vi "paths.vi"() -> ()   [LabVIEW 2022 SP3]
uses:
  <vilib>/Utility/file.llb/Write Delimited Spreadsheet (string).vi
panel:
  out "Array 2":path[](array[path])
  out "filenames":string[][](array[string])
  in  "path":path=path "D:/Doppler Retro/2009"
  in  "folder names 2":string[](array[string])
  out "Array":path[](array[path])
  out "folder names":string[](array[string])
  out "All Files in Dir":path[](array[path])
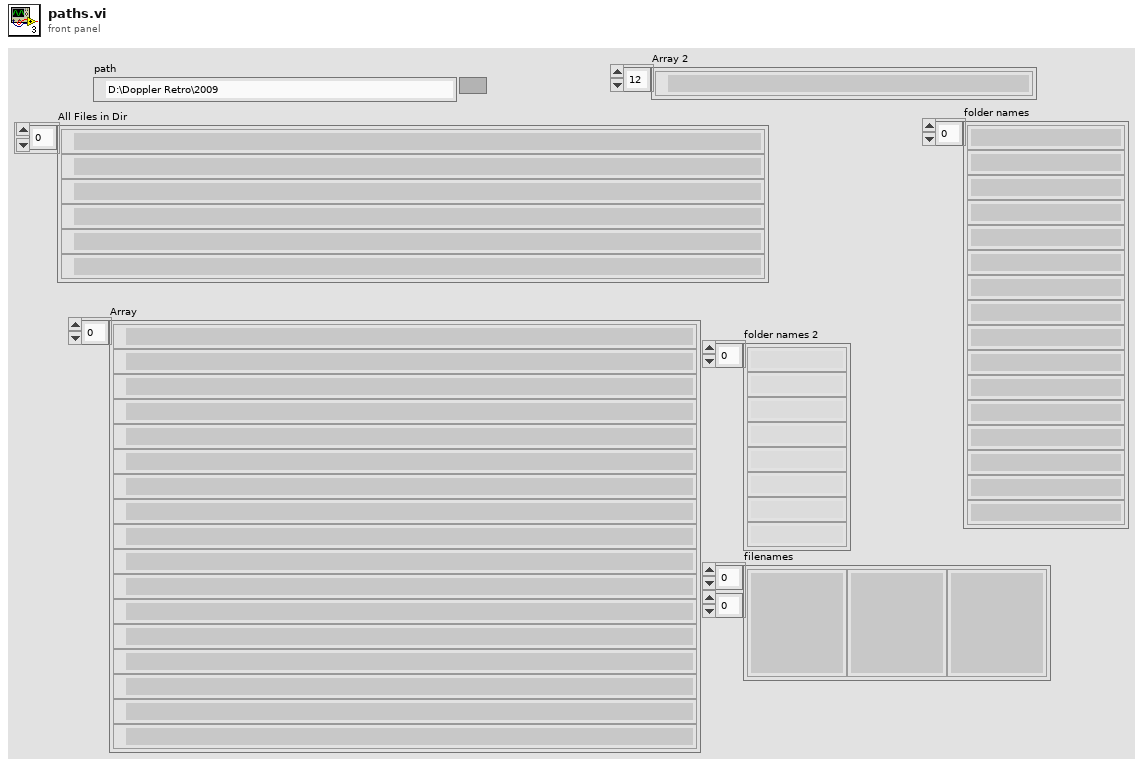
[diagram p1: front panel]
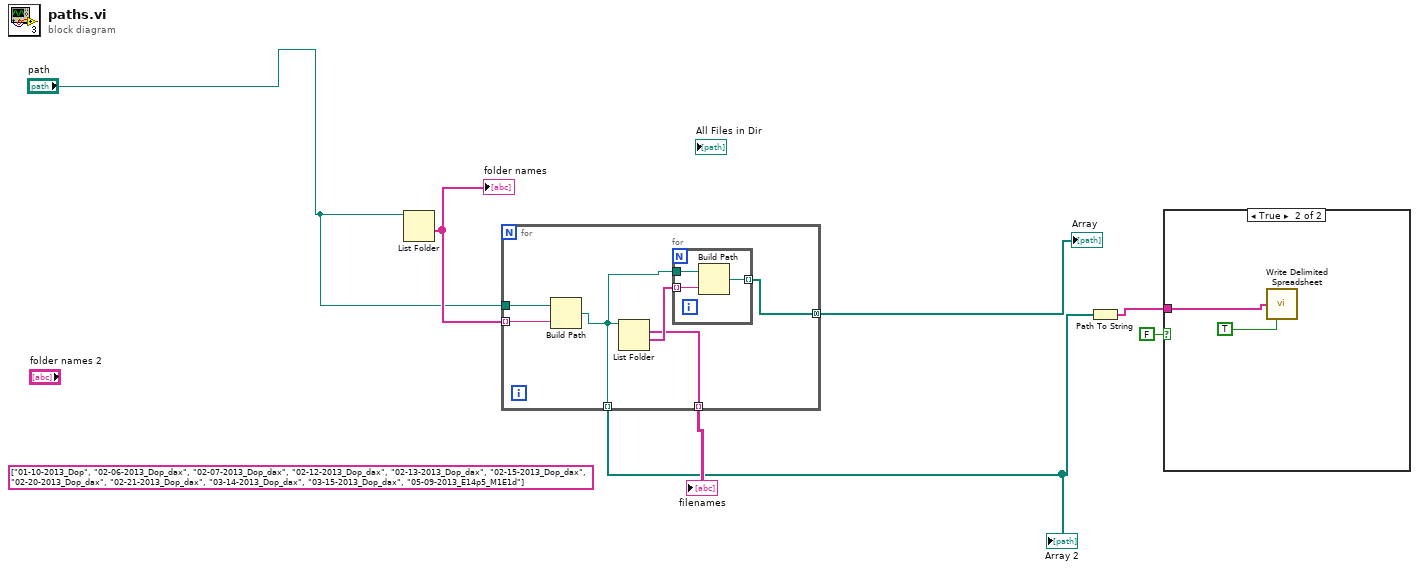
[diagram p0: block diagram]
diagram:
  (unwired) string[] ["01-10-2013_Dop", "02-06-2013_Dop_dax", "02-07-2013_Dop_dax", "02-12-2013_Dop_dax", "02-13-2013_Dop_dax", "02-15-2013_Dop_dax", "02-20-2013_Dop_dax", "02-21-2013_Dop_dax", "03-14-2013_Dop_dax", "03-15-2013_Dop_dax", "05-09-2013_E14p5_M1E1d"] ("folder names")
  n1 = List Folder(path="path") -> (folder names=w4:string[])  [unwired: 3 in, 3 out]
  "folder names" <- w4
  n2 = for {
    tunnel: "path" -> [w13]
    tunnel: w4 -> [w12] mode=indexing
    tunnel: [w10] -> w7 mode=concatenating
    tunnel: [w9] -> w2 mode=indexing
    tunnel: [w8] -> w1 mode=indexing
    n3 = Build Path(base path=w13, name or relative path=w12) -> (appended path=w8:path)
    n4 = List Folder(path=w8) -> (filenames=w9:string[], folder names=w11:string[])  [unwired: 3 in, 2 out]
    n5 = for {
      tunnel: w8 -> [w16]
      tunnel: w11 -> [w15] mode=indexing
      tunnel: [w14] -> w10 mode=indexing
      n6 = Build Path(base path=w16, name or relative path=w15) -> (appended path=w14:path)
    }
  }
  "Array" <- w7
  "filenames" <- w2
  "Array 2" <- w1
  n7 = Path To String(path=w1) -> (string=w6:string[])
  n8 = case shown="True" FALSE {
    tunnel: w6 -> [_ w17]
    frame False {
    }
    frame True {
      n9 = call-poly <vilib>:"Write Delimited Spreadsheet.vi"("1D data"=w17, "transpose? (no:F)"=TRUE) -> ()  [unwired: 12 in, 2 out]
    }
  }
